vi "dBData-ParseDataToUpdate.vi"(0 "ERP-SpecificationManager in":refnum<class "ERP-SpecificationManager.lvclass">, 11 "error in (no error)":errorcluster) -> (3 "SQL Statement":string, 4 "ERP-SpecificationManager out":refnum<class "ERP-SpecificationManager.lvclass">, 8 "Payload":string, 10 "Column":i32, 15 "error out":errorcluster)   [LabVIEW 2013, in "ERP-SpecificationManager.lvclass"]
uses:
  ERP-SpecificationManager.lvclass
  ERP-SpecificationManager.lvclass/ERP-SpecificationManager.ctl
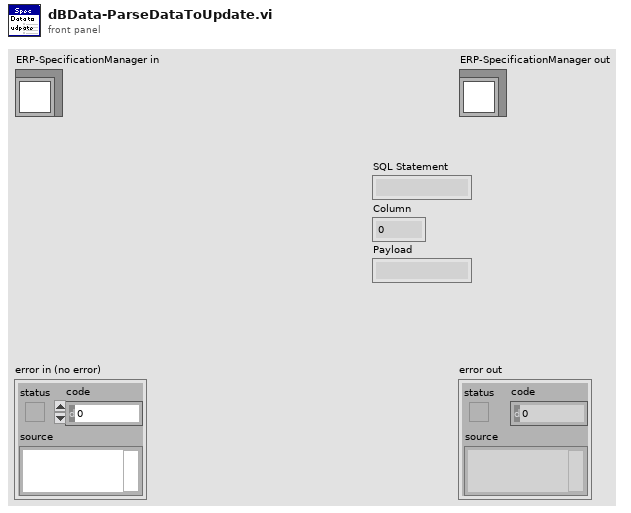
[diagram p1: front panel]
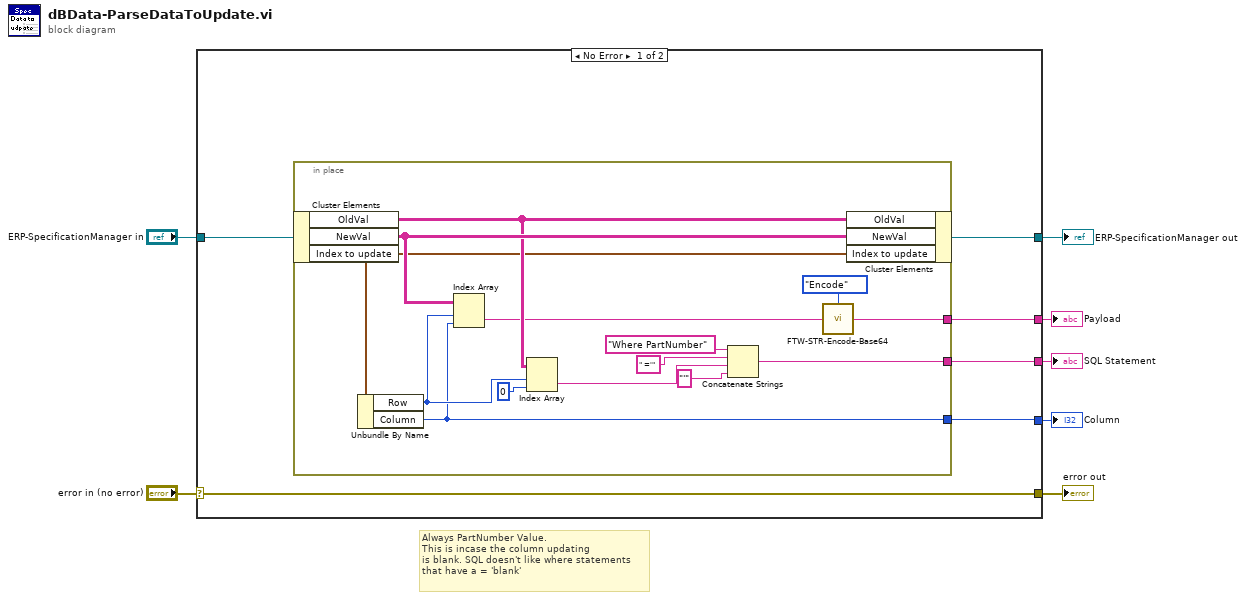
[diagram p0: block diagram]
diagram:
  # "Always PartNumber Value. \nThis is incase the column updating\nis blank. SQL doesn't like where statements\nthat have a = 'blank'"
  n1 = case shown="No Error" "error in (no error)" {
    selector: "error in (no error)" -> [w13 w29]
    tunnel: [w13 w29] -> w6
    tunnel: [w11 w28] -> w4
    tunnel: "ERP-SpecificationManager in" -> [w12 w28]
    tunnel: [w10 _] -> w3
    tunnel: [w9 _] -> w2
    tunnel: [w8 _] -> w1
    frame No Error {
      n2 = in-place {
        in-place-border: [w18] -> w10
        in-place-border: [w17] -> w9
        in-place-border: [w14] -> w8
        n3 = in-place-cluster #1(w12) -> ("OldVal"=w24:string[][], "NewVal"=w25:string[][], "Index to update"=w23:cluster{"Column":i32, "Row":i32})
        n4 = Unbundle By Name(w23) -> ("Row"=w26:i32, "Column"=w17:i32)
        n5 = Index Array(array=w25, index (row)=w26, index (col)=w17) -> (element=w15:string)
        n6 = Index Array(array=w24, index (row)=w26, index (col)=0 ("disabled index (col)")) -> (element=w19:string)
        n7 = Concatenate Strings("Where PartNumber" ("condition"), " ='" ("condition"), w19, "'" ("string")) -> (w18:string)
        n8 = call "FTW-STR-Encode-Base64.vi"("Input"=w15, "Direction"=enum16{"Encode", "Decode"}."Encode") -> ("Output"=w14:string)
        n9 = in-place-cluster #1("OldVal"=w24, "NewVal"=w25, "Index to update"=w23) -> (w11:refnum<class "ERP-SpecificationManager.lvclass">)
      }
    }
    frame Error {
    }
  }
  "error out" <- w6
  "ERP-SpecificationManager out" <- w4
  "SQL Statement" <- w3
  "Column" <- w2
  "Payload" <- w1
